vi "Grating.vi"(11 "General settings":T1) -> (2 "grating":dbl[][](array[numeric]))   [LabVIEW 2014]
uses:
  Controls/SLM General Settings.ctl
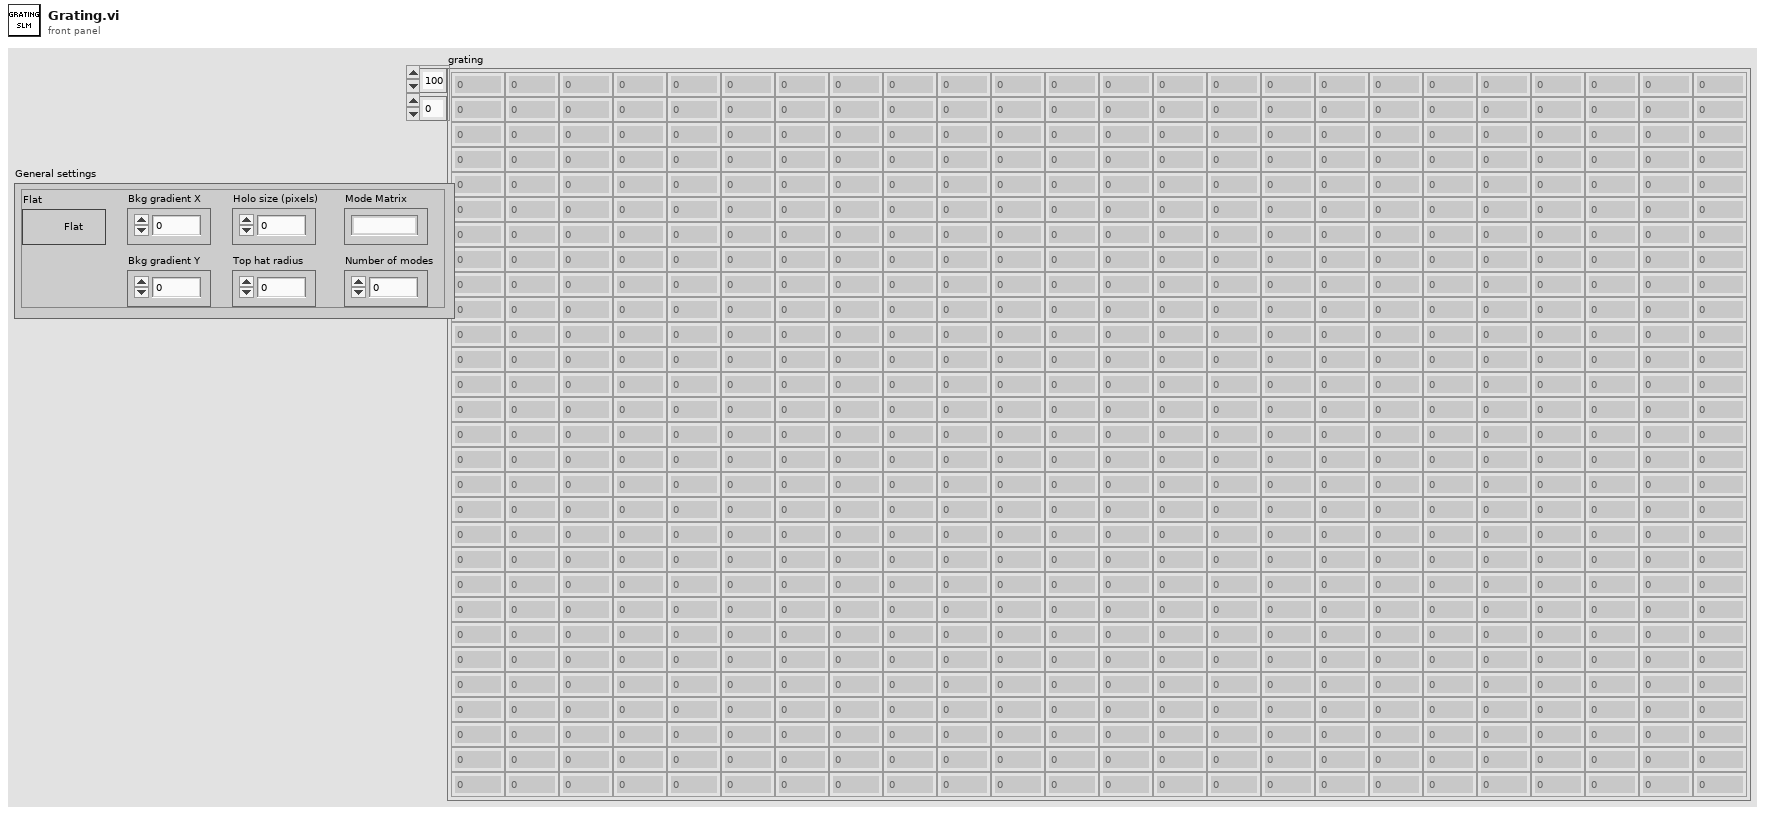
[diagram p1: front panel]
types:
  T1 = typedef "SLM General Settings.ctl" = cluster{"Holo size (pixels)":i32, "Top hat radius":dbl, "Number of modes":i32, "Bkg gradient X":dbl, "Bkg gradient Y":dbl, "Flat":bool, "Mode Matrix":u16}
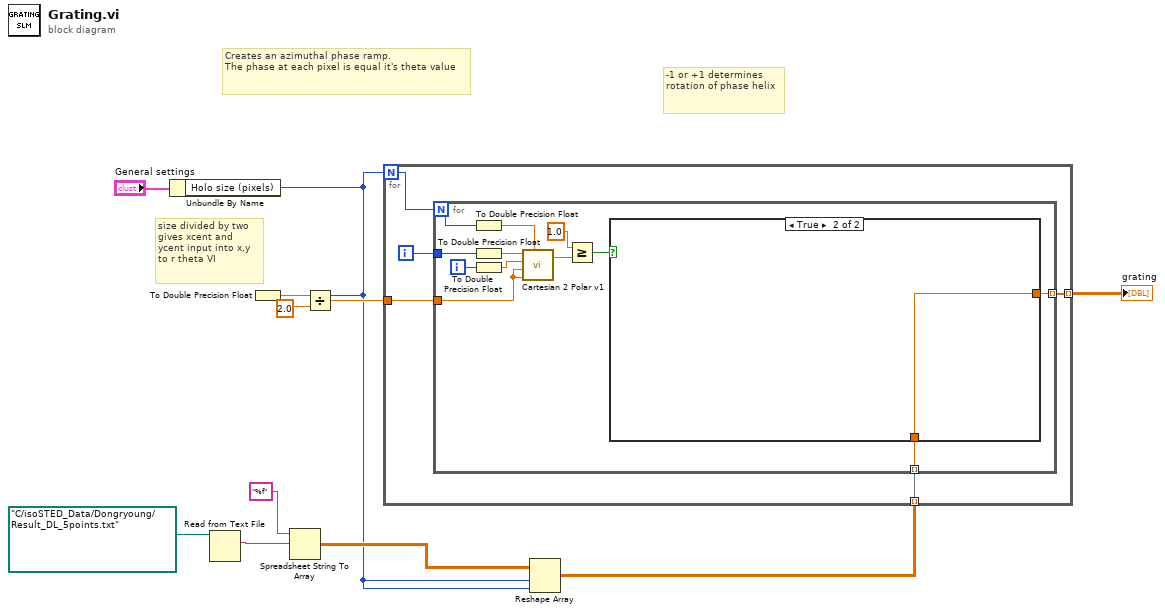
[diagram p0: block diagram]
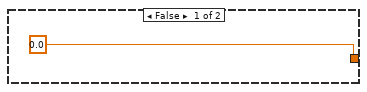
[diagram p2: hidden frame]
diagram:
  # "-1 or +1 determines \nrotation of phase helix"
  # "Creates an azimuthal phase ramp.\nThe phase at each pixel is equal it's theta value"
  # "size divided by two gives xcent and ycent input into x,y to r theta VI"
  n1 = Unbundle By Name("General settings") -> ("Holo size (pixels)"=w3:i32)
  n2 = Read from Text File(file (use dialog)=path "C:/isoSTED_Data/Dongryoung/Result_DL_5points.txt" ("file (use dialog) 2")) -> (text=w5:string)  [unwired: 3 in, 3 out]
  n3 = To Double Precision Float(number=w3) -> (double precision float=w8:dbl)
  n4 = Spreadsheet String To Array(format string="%f", spreadsheet string=w5) -> (array=w4:dbl[][])  [unwired: 2 in]
  n5 = Divide(x=w8, y=2.0) -> (x/y=w11:dbl)
  n6 = Reshape Array(w4, w3, w3) -> (w2:dbl[][])
  n7 = for {
    N: w3 -> [w14]
    tunnel: w11 -> [w15]
    tunnel: [w13] -> w1 mode=indexing
    tunnel: w2 -> [w12] mode=indexing
    i -> [w16]
    n8 = for {
      N: w14 -> [w19]
      tunnel: w16 -> [w20]
      tunnel: w15 -> [w25]
      tunnel: [w18] -> w13 mode=indexing
      tunnel: w12 -> [w17] mode=indexing
      i -> [w21]
      n9 = To Double Precision Float(number=w19) -> (double precision float=w24:dbl)
      n10 = To Double Precision Float(number=w20) -> (double precision float=w23:dbl)
      n11 = To Double Precision Float(number=w21) -> (double precision float=w22:dbl)
      n12 = call "Cartesian 2 Polar v1.vi"("x"=w23, "y"=w22, "xcent"=w25, "ycent"=w25, "diam"=w24) -> ("r"=w27:dbl)  [unwired: 1 out]
      n13 = Greater Or Equal?(x=1.0, y=w27) -> (x >= y?=w28:bool)
      n14 = case shown="True" w28 {
        tunnel: [0.0 ("zernike") w30] -> w18
        tunnel: w17 -> [_ w30]
        frame False {
        }
        frame True {
        }
      }
    }
  }
  "grating" <- w1
